vi "Option Knobs.vi"(7 "Standalone?":bool, 8 "Error In":errorcluster, 10 "Option Knobs":T2(ring)=enum."OptionKnob2Position2", 11 "GEA2 Reference In":refnum<k24>) -> (0 "Error Out":errorcluster, 3 "GEA2 Reference Out":refnum<k24>)   [LabVIEW 2016, in "Centauro.lvlib"]
uses:
  Projects/Centauro.lvlib
  Q:/Common/DLLs/GEA3/GeaCommunication.dll
  Common/DLLs/GEA3/GeaCommunication.dll
  Tools/Laundry/Centauro Tool/Centauro Tool Support/type defs/Event Sequence.ctl
  Common/LabVIEW GEA2 Toolkit/LabVIEW_GEA2_Toolkit.lvlibp/type defs/Source_Destination.ctl
  Common/LabVIEW GEA2 Toolkit/LabVIEW_GEA2_Toolkit.lvlibp
panel:
  in  "Event ID":T1
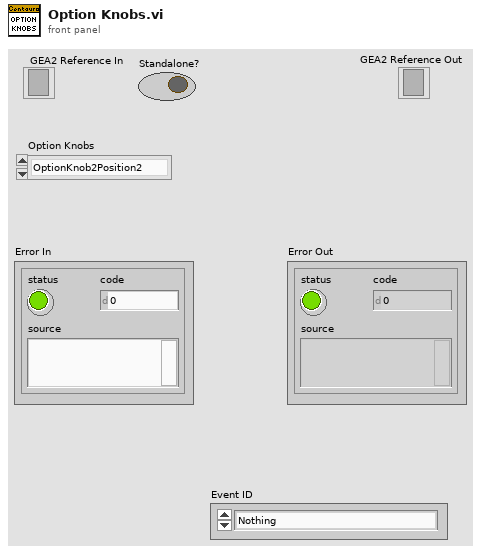
[diagram p1: front panel]
types:
  T1 = typedef "Event Sequence.ctl" = enum16{"Nothing", "StartButtonPress", "StartButtonRelease", "DeepRinseKeyPress", "DeepRinseKeyRelease", "CycleKnobPosition0", "CycleKnobPosition1", "CycleKnobPosition2", "CycleKnobPosition3", "CycleKnobPosition4", "CycleKnobPosition5", "CycleKnobPosition6", "CycleKnobPosition7", "CycleKnobPosition8", "CycleKnobPosition9", "CycleKnobPosition10", "CycleKnobPosition11", "OptionKnob1Position0", "OptionKnob1Position1", "OptionKnob1Position2", "OptionKnob1Position3", "OptionKnob1Position4", "OptionKnob1Position5", "OptionKnob2Position0", "OptionKnob2Position1", "OptionKnob2Position2", "OptionKnob2Position3", "OptionKnob2Position4"}
  T2 = enum16{"OptionKnob1Position0", "OptionKnob1Position1", "OptionKnob1Position2", "OptionKnob1Position3", "OptionKnob1Position4", "OptionKnob1Position5", "OptionKnob2Position0", "OptionKnob2Position1", "OptionKnob2Position2", "OptionKnob2Position3", "OptionKnob2Position4"}
  T3 = typedef "LabVIEW_GEA2_Toolkit.lvlibp/Source_Destination.ctl" = cluster{"Source":u8, "Destination":u8}
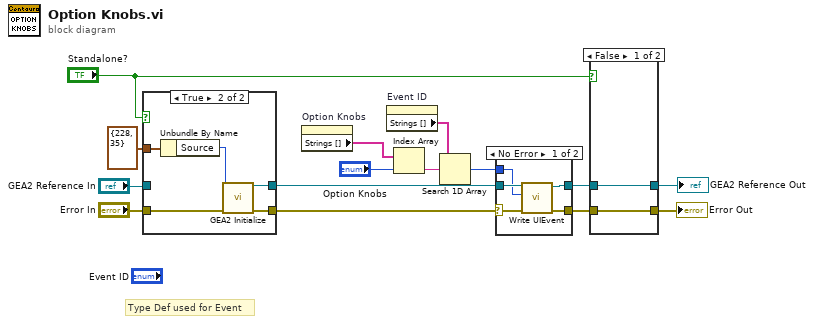
[diagram p0: block diagram]
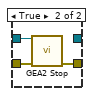
[diagram p2: hidden frame]
diagram:
  # "Type Def used for Event"
  n1 = case shown="True" "Standalone?" {
    tunnel: "Error In" -> [w16 w22]
    tunnel: [w16 w21] -> w2
    tunnel: "GEA2 Reference In" -> [w17 _]
    tunnel: [w17 w20] -> w1
    tunnel: T3 {"Source"=228, "Destination"=35} ("GEA Inputs") -> [_ w18]
    frame False {
    }
    frame True {
      n2 = Unbundle By Name(w18) -> ("Source"=w19:u8)
      n3 = call "GEA2 Initialize.vi"("Source Address"=w19, "error in"=w22) -> ("GEA2 Reference Out"=w20:refnum<k24>, "error out"=w21:errorcluster)  [unwired: 11 in, 1 out]
    }
  }
  n4 = property on="Option Knobs" class="Enum (strict)"() -> ("Strings []"=w15:string[])  [unwired: 2 in, 2 out]
  n5 = property on="Event ID" class="Enum (strict)"() -> ("Strings []"=w13:string[])  [unwired: 2 in, 2 out]
  n6 = Index Array(array=w15, index="Option Knobs") -> (element=w12:string)
  n7 = Search 1D Array(1D array=w13, element=w12) -> (index of element=w11:i32)  [unwired: 1 in]
  n8 = case shown="No Error" w2 {
    selector: w2 -> [w26 w29]
    tunnel: [w27 w29] -> w8
    tunnel: w1 -> [w25 w28]
    tunnel: [w24 w28] -> w9
    tunnel: w11 -> [w23 _]
    frame No Error {
      n9 = call "Write UIEvent.vi"("Error In"=w26, "Event ID"=w23, "GEA2 Reference In"=w25) -> ("Error Out"=w27:errorcluster, "GEA2 Reference Out"=w24:refnum<k24>)  [unwired: 7 in]
    }
    frame Error {
    }
  }
  n10 = case shown="False" "Standalone?" {
    tunnel: [w30 w34] -> w6
    tunnel: w9 -> [w31 w33]
    tunnel: [w31 _] -> w7
    tunnel: w8 -> [w30 w32]
    frame False {
    }
    frame True {
      n11 = call "GEA2 Stop.vi"("GEA2 Reference In"=w33, "Error In"=w32) -> ("Error Out"=w34:errorcluster)  [unwired: 13 in]
    }
  }
  "Error Out" <- w6
  "GEA2 Reference Out" <- w7
